vi "数据入队.vi"(1 "新元素/子数组":dbl, 2 "源数组":dbl[](array[numeric])) -> (0 "已删除元素的数组子集":dbl[](array[numeric]))   [LabVIEW 2018]
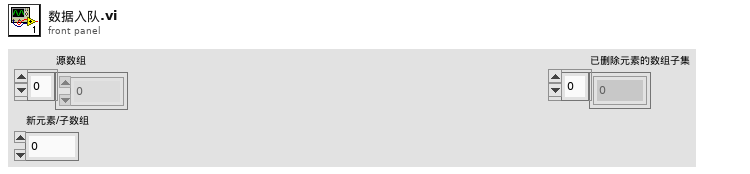
[diagram p1: front panel]
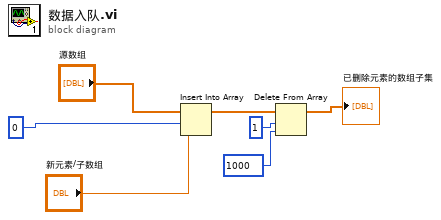
[diagram p0: block diagram]
diagram:
  n1 = Insert Into Array(array="源数组", index=0 ("索引"), new element="新元素/子数组") -> (w4:dbl[])
  n2 = Delete From Array(array=w4, length=1 ("长度"), index=1000 ("索引")) -> (array with subset deleted=→"已删除元素的数组子集":dbl[])  [unwired: 1 out]
